vi "ContFindAcquisition.vi"(11 "ItemNames":string[][](array[string])) -> (3 "Array":i32[][](array[numeric]))   [LabVIEW 2018, in "Config.lvlib"]
uses:
  Config/Config.lvlib
  <vilib>/regexp/Match Regular Expression.xnode
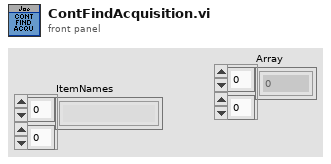
[diagram p1: front panel]
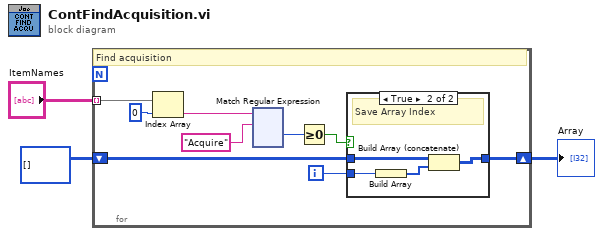
[diagram p0: block diagram]
diagram:
  n1 = for {
    shift-right: [w9] -> w2
    shift-left: i32[][] [] -> [w8]
    tunnel: "ItemNames" -> [w5] mode=indexing
    i -> [w4]
    # "Find acquisition"
    n2 = Index Array(array=w5, index=0 ("disabled index (col)")) -> (element=w7:string)
    n3 = xnode "Match Regular Expression"("input string"=w7, "regular expression"="Acquire" ("element")) -> ("offset past match"=w11:i32)  [unwired: 4 in, 4 out]
    n4 = Greater Or Equal To 0?(x=w11) -> (x >= 0?=w10:bool)
    n5 = case shown="True" w10 {
      tunnel: [w13 w17] -> w9
      tunnel: w8 -> [w13 w16]
      tunnel: w4 -> [_ w14]
      frame False {
      }
      frame True {
        # "Save Array Index"
        n6 = Build Array(w14) -> (w15:i32[])
        n7 = Build Array (concatenate)(w16, w15) -> (w17:i32[][])
      }
    }
  }
  "Array" <- w2
